vi "Create Assembly config file.vi"() -> ()   [LabVIEW 2023]
uses:
  Source/EIP Attribute Configuration.ctl
  Source/EIP Attribute Direction.ctl
  Source/Ethernet IP Custom Device Custom Device.lvlib
panel:
  out "error out":errorcluster
  in  "file (use dialog)":path=path "C:/git/fmussi_Ethernet-IP-Custom-Device/Tests/TestAssemblyConfig.csv"
  in  "Config":T1[](array[typedef])=[{"Name"="a", "Direction"=enum."Input", "Class"=1, "Instance"=0, "Attribute"=100, "size in bytes"=4}, {"Name"="b", "Direction"=enum."Input", "Class"=1, "Instance"=1, "Attribute"=101, "size in bytes"=4}, {"Name"="c", "Direction"=enum."Input", "Class"=1, "Instance"=2, "Attribute"=102, "size in bytes"=4}, {"Name"="d", "Direction"=enum."Output", "Class"=2, "Instance"=3, "Attribute"=103, "size in bytes"=4}, {"Name"="e", "Direction"=enum."Output", "Class"=2, "Instance"=4, "Attribute"=104, "size in bytes"=4}, {"Name"="f", "Direction"=enum."Output", "Class"=2, "Instance"=5, "Attribute"=105, "size in bytes"=4}]
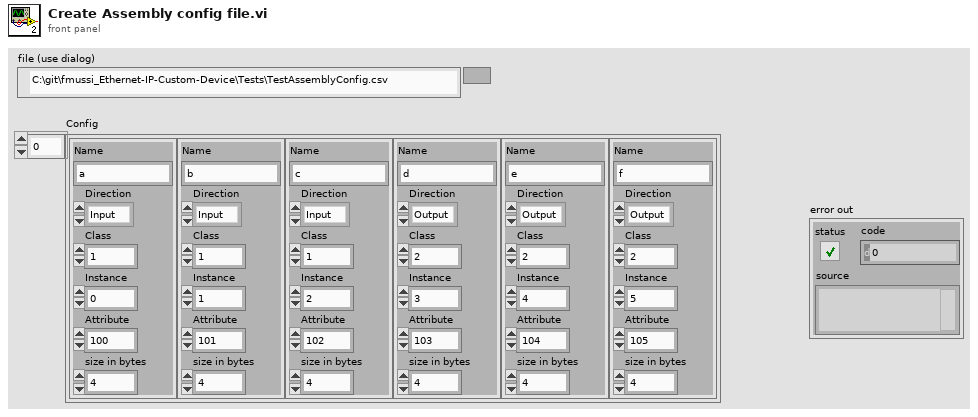
[diagram p1: front panel]
types:
  T1 = typedef "Ethernet IP Custom Device Custom Device.lvlib/EIP Attribute Configuration.ctl" = cluster{"Name":string, "Direction":T2, "Class":i32, "Instance":u32, "Attribute":i32, "size in bytes":i32}
  T2 = typedef "Ethernet IP Custom Device Custom Device.lvlib/EIP Attribute Direction.ctl" = enum16{"Input", "Output"}
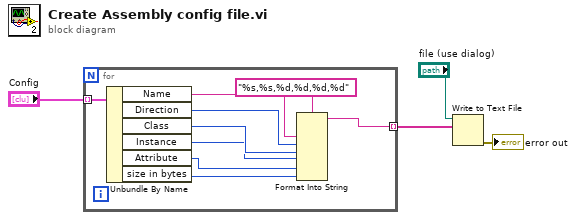
[diagram p0: block diagram]
diagram:
  n1 = for {
    tunnel: "Config" -> [w13] mode=indexing
    tunnel: [w7] -> w3 mode=indexing
    n2 = Unbundle By Name(w13) -> ("Name"=w6:string, "Direction"=w5:T2, "Class"=w12:i32, "Instance"=w11:u32, "Attribute"=w10:i32, "size in bytes"=w9:i32)
    n3 = Format Into String(format string="%s,%s,%d,%d,%d,%d", w6, w5, w12, w11, w10, w9) -> (resulting string=w7:string)  [unwired: 2 in, 1 out]
  }
  n4 = Write to Text File(file (use dialog)="file (use dialog)", text=w3) -> (error out=→"error out":errorcluster)  [unwired: 2 in, 2 out]
